vi "Add.vi"(10 "y":dbl, 11 "x":dbl) -> (2 "x+y+z":dbl)   [LabVIEW 2017]
panel:
  in  "z":dbl
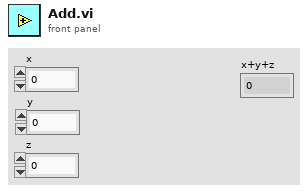
[diagram p1: front panel]
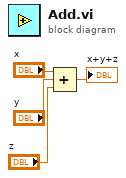
[diagram p0: block diagram]
diagram:
  n1 = Compound Arithmetic op=ADD("x", "y", "z") -> (→"x+y+z":dbl)
